vi "Лабораторная №1 Задание 3_6.vi"() -> ()   [LabVIEW 2017]
panel:
  out "Полных часов осталось":dbl
  out "Оставшееся время, мин":dbl
  in  "ММ":dbl min=0.0 max=60.0 step=1.0
  in  "ЧЧ":dbl min=0.0 max=24.0 step=1.0
  in  "ММ":dbl min=0.0 max=60.0 step=1.0
  in  "ЧЧ":dbl min=0.0 max=24.0 step=1.0
  # "Текущее время"
  # "Конечное время"
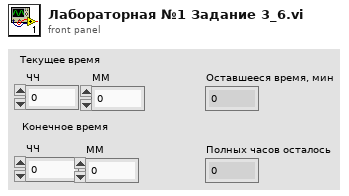
[diagram p1: front panel]
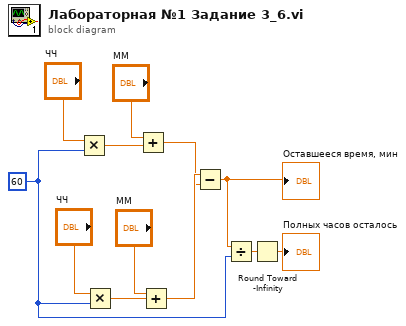
[diagram p0: block diagram]
diagram:
  w4 = 60
  n1 = Multiply(x="ЧЧ", y=w4) -> (x*y=w10:dbl)
  n2 = Multiply(x="ЧЧ", y=w4) -> (x*y=w8:dbl)
  n3 = Add(x="ММ", y=w10) -> (x+y=w5:dbl)
  n4 = Add(x="ММ", y=w8) -> (x+y=w6:dbl)
  n5 = Subtract(x=w6, y=w5) -> (x-y=w3:dbl)
  "Оставшееся время, мин" <- w3
  n6 = Divide(x=w3, y=w4) -> (x/y=w2:dbl)
  n7 = Round Toward -Infinity(1:w2) -> (0:→"Полных часов осталось":dbl)
